vi "Parse Crowbar Fault.vi"(11 "Crowbar Fault":u8 format="%02x") -> (3 "Crowbar":T1 {"Crowbar Fault" format="%02x"})   [LabVIEW 2020]
uses:
  Crowbar Display.ctl
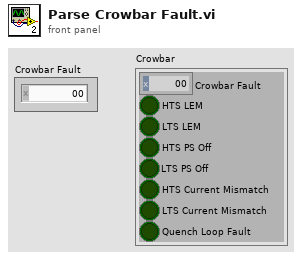
[diagram p1: front panel]
types:
  T1 = typedef "Crowbar Display.ctl" = cluster{"Crowbar Fault":u8, "HTS LEM":bool, "LTS LEM":bool, "HTS PS Off":bool, "LTS PS Off":bool, "HTS Current Mismatch":bool, "LTS Current Mismatch":bool, "Quench Loop Fault":bool}
  T2 = cluster{"Crowbar Fault":u8, bool, bool, bool, bool, bool, bool, bool}
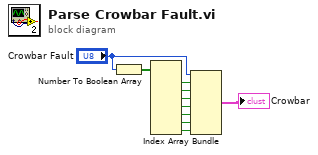
[diagram p0: block diagram]
diagram:
  n1 = Number To Boolean Array(number="Crowbar Fault") -> (Boolean array=w9:bool[])
  n2 = Index Array(array=w9) -> (element #1=w7:bool, element #2=w6:bool, element #3=w5:bool, element #4=w4:bool, element #5=w3:bool, element #6=w2:bool, element #7=w1:bool)  [unwired: 7 in]
  n3 = Bundle("Crowbar Fault"="Crowbar Fault", w7, w6, w5, w4, w3, w2, w1) -> (→"Crowbar":T2)  [unwired: 1 in]
